vi "Nodes.vi"(7 "LabVIEW Web Service Request":refnum<class "Web Request.lvclass">) -> ()   [LabVIEW 2021]
uses:
  <vilib>/wsapi/Web Request.lvclass
  <vilib>/GPower/String v2/Library/String v2.lvlib
panel:
  out "array":string[](array[string])
  out "Occurrences":i32[](array[numeric])
  out "Type":string
  out "request variables":cluster{"Key":string[], "Value":string[]}
  out "value":string
  # "Use the Web Service Request input terminal to call the VIs on the Web Services palette. Do not remove it from the connector pane unless you don't need access to the palette."
  # "Each additional control wired to the connector pane will be available as an input in the URL. To include an indicator in terminal-mode output (the default setting), it must also be wired to the connector pane."
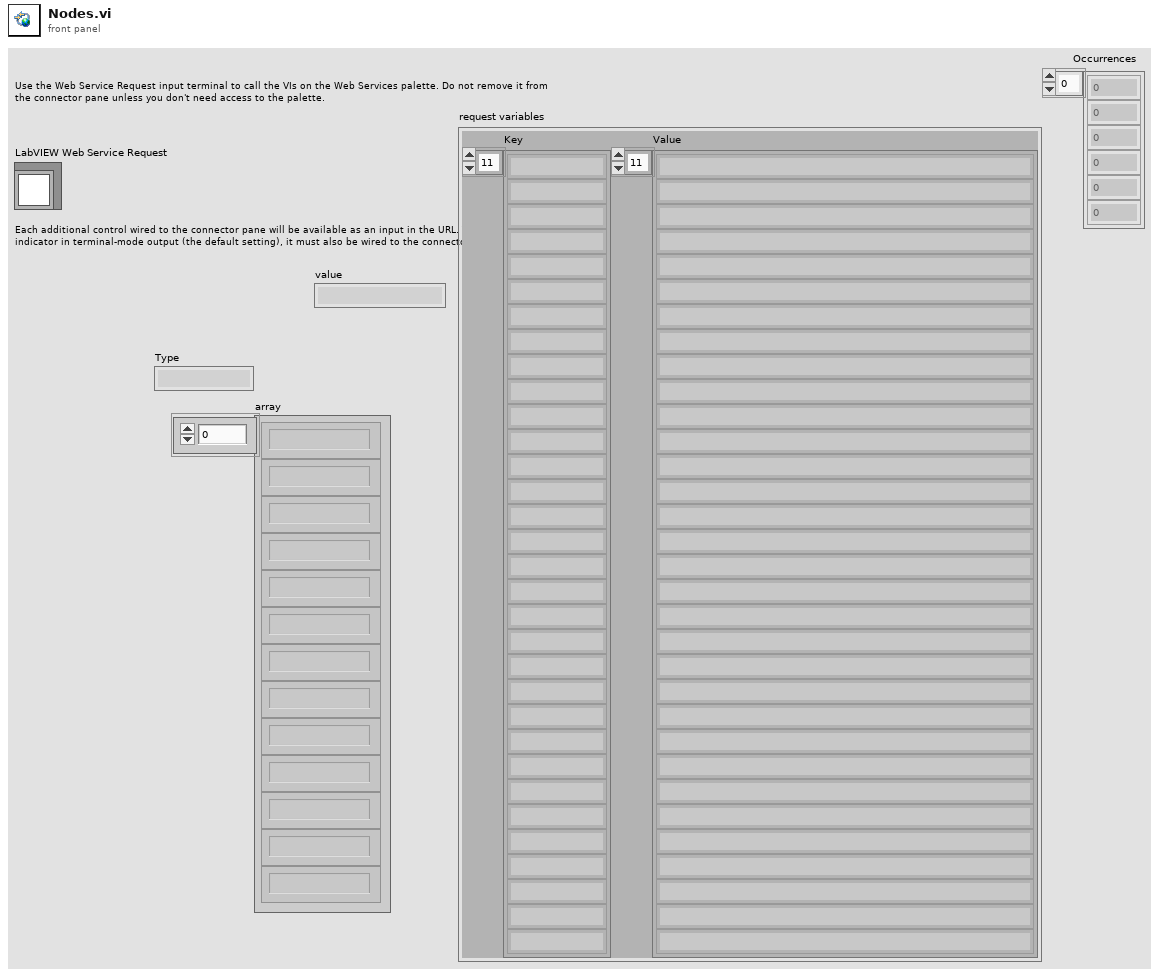
[diagram p1: front panel]
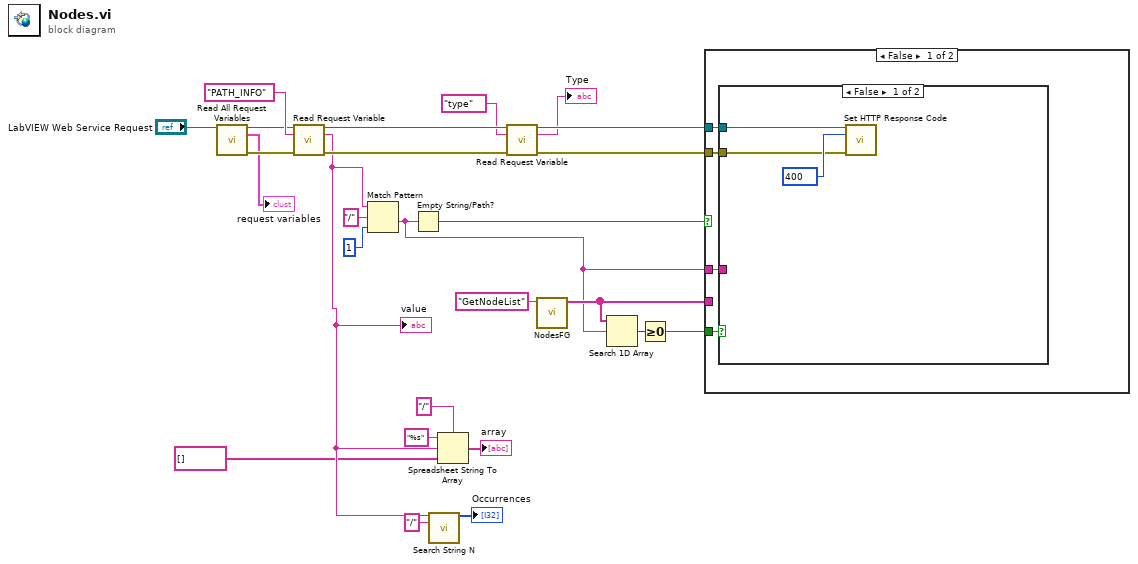
[diagram p0: block diagram]
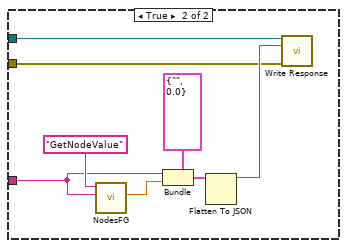
[diagram p2: hidden frame]
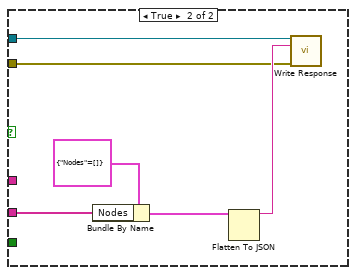
[diagram p3: hidden frame]
diagram:
  n1 = call <vilib>:"Read All Request Variables.vi"("LabVIEW Web Service Request"="LabVIEW Web Service Request") -> ("LabVIEW Web Service Request out"=w24:refnum<class "Web Request.lvclass">, "request variables"=→"request variables":cluster{"Key":string[], "Value":string[]}, "error out"=w23:errorcluster)  [unwired: 12 in]
  n2 = call <vilib>:"Read Request Variable.vi"("LabVIEW Web Service Request"=w24, "variable name"="PATH_INFO", "error in (no error)"=w23) -> ("LabVIEW Web Service Request out"=w12:refnum<class "Web Request.lvclass">, "value"=w5:string, "error out"=w13:errorcluster)  [unwired: 10 in]
  "value" <- w5
  n3 = Match Pattern(string=w5, regular expression="/", offset (0)=1) -> (after substring=w15:string)  [unwired: 3 out]
  n4 = Empty String/Path?(string/path=w15) -> (empty?=w18:bool)
  n5 = call <vilib>:"Search String N.vi"("String"=w5, "Search String"="/") -> ("Occurrences"=→"Occurrences":i32[])  [unwired: 13 in]
  n6 = Spreadsheet String To Array(delimiter (Tab)="/", format string="%s", spreadsheet string=w5, array type (2D Dbl)=string[] []) -> (array=→"array":string[])
  n7 = call <vilib>:"Read Request Variable.vi"("LabVIEW Web Service Request"=w12, "variable name"="type", "error in (no error)"=w13) -> ("LabVIEW Web Service Request out"=w11:refnum<class "Web Request.lvclass">, "value"=→"Type":string, "error out"=w10:errorcluster)  [unwired: 10 in]
  n8 = call "NodesFG.vi"("Function"="GetNodeList") -> ("Node List"=w16:string[])  [unwired: 8 in, 2 out]
  n9 = Search 1D Array(1D array=w16, element=w15) -> (index of element=w17:i32)  [unwired: 1 in]
  n10 = Greater Or Equal To 0?(x=w17) -> (x >= 0?=w14:bool)
  n11 = case shown="False" w18 {
    tunnel: w16 -> [_ w46]
    tunnel: w15 -> [w30 _]
    tunnel: w14 -> [w29 _]
    tunnel: w10 -> [w28 w42]
    tunnel: w11 -> [w27 w43]
    frame False {
      n12 = case shown="False" w29 {
        tunnel: w30 -> [_ w40]
        tunnel: w28 -> [w31 w34]
        tunnel: w27 -> [w32 w35]
        frame False {
          w33 = 400 items=["100"=100, "101"=101, "200"=200, "201"=201, "202"=202, "203"=203, "204"=204, "205"=205, "206"=206, "300"=300, "301"=301, "302"=302, "303"=303, "304"=304, "305"=305, "306"=306, "307"=307, "400"=400, "401"=401, "402"=402, "403"=403, "404"=404, "405"=405, "406"=406, "407"=407, "408"=408, "409"=409, "410"=410, "411"=411, "412"=412, "413"=413, "414"=414, "415"=415, "416"=416, "417"=417, "500"=500, "501"=501, "502"=502, "503"=503, "504"=504, "505"=505] ("response code (200)")
          n13 = call <vilib>:"Set HTTP Response Code.vi"("LabVIEW Web Service Request"=w32, "response code (200)"=w33, "error in (no error)"=w31) -> ()  [unwired: 11 in, 2 out]
        }
        frame True {
          n14 = call "NodesFG.vi"("Node Name"=w40, "Function"="GetNodeValue") -> ("Value"=w39:dbl)  [unwired: 7 in, 2 out]
          n15 = Bundle(cluster=cluster{"name":string, "Value":dbl} {"name"="", "Value"=0.0}, "name"=w40, "Value"=w39) -> (w37:cluster{"name":string, "Value":dbl})
          n16 = Flatten To JSON(anything=w37) -> (JSON string=w36:string)  [unwired: 2 in, 1 out]
          n17 = call <vilib>:"Write Response.vi"("LabVIEW Web Service Request"=w35, "response string"=w36, "error in (no error)"=w34) -> ()  [unwired: 11 in, 2 out]
        }
      }
    }
    frame True {
      n18 = Bundle By Name(cluster=cluster{"Nodes":string[]} {"Nodes"=[]}, "Nodes"=w46) -> (w45:cluster{"Nodes":string[]})
      n19 = Flatten To JSON(anything=w45) -> (JSON string=w44:string)  [unwired: 2 in, 1 out]
      n20 = call <vilib>:"Write Response.vi"("LabVIEW Web Service Request"=w43, "response string"=w44, "error in (no error)"=w42) -> ()  [unwired: 11 in, 2 out]
    }
  }
